vi "Flow_Sensor_Filter_subVI.vi"(10 "Apply dF/dt?":bool, 11 "Flow Rate Data Out":cluster{dbl, dbl, dbl, dbl, dbl}) -> (3 "Cluster":T1)   [LabVIEW 2015]
uses:
  <vilib>/ptbypt/NI_PtbyPt.lvlib
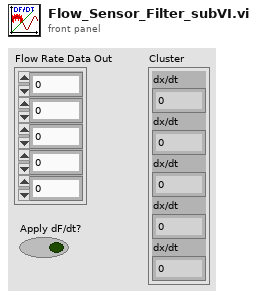
[diagram p1: front panel]
types:
  T1 = cluster{"dx/dt":dbl, "dx/dt":dbl, "dx/dt":dbl, "dx/dt":dbl, "dx/dt":dbl}
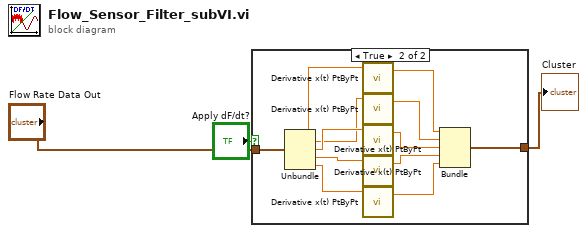
[diagram p0: block diagram]
diagram:
  n1 = case shown="True" "Apply dF/dt?" {
    tunnel: "Flow Rate Data Out" -> [_ w15]
    tunnel: [_ w4] -> w3
    frame False {
    }
    frame True {
      n2 = Unbundle(w15) -> (w10:dbl, w11:dbl, w12:dbl, w13:dbl, w14:dbl)
      n3 = call <vilib>:"Derivative x(t) PtByPt.vi"("x"=w10) -> ("dx/dt"=w5:dbl)  [unwired: 3 in, 1 out]
      n4 = call <vilib>:"Derivative x(t) PtByPt.vi"("x"=w11) -> ("dx/dt"=w6:dbl)  [unwired: 3 in, 1 out]
      n5 = call <vilib>:"Derivative x(t) PtByPt.vi"("x"=w12) -> ("dx/dt"=w7:dbl)  [unwired: 3 in, 1 out]
      n6 = call <vilib>:"Derivative x(t) PtByPt.vi"("x"=w13) -> ("dx/dt"=w8:dbl)  [unwired: 3 in, 1 out]
      n7 = call <vilib>:"Derivative x(t) PtByPt.vi"("x"=w14) -> ("dx/dt"=w9:dbl)  [unwired: 3 in, 1 out]
      n8 = Bundle("dx/dt"=w5, "dx/dt"=w6, "dx/dt"=w7, "dx/dt"=w8, "dx/dt"=w9) -> (w4:T1)  [unwired: 1 in]
    }
  }
  "Cluster" <- w3
